vi "3phase PLL.vi"(0 "A":fxp<+/-,32,4>, 1 "wo":dbl, 2 "B":fxp<+/-,32,4>, 3 "C":fxp<+/-,32,4>, 4 "dt (s)":dbl=-1.0 format="%.3f", 5 "PID gains":T1={"proportional gain (Kc)"=1.0, "integral time (Ti, min)"=0.01, "derivative time (Td, min)"=0.0} {"derivative time (Td, min)" format="%.3f"; "integral time (Ti, min)" format="%.3f"; "proportional gain (Kc)" format="%.3f"}) -> (6 "Frequency":dbl, 7 "Phase":dbl)   [LabVIEW 2016]
uses:
  <vilib>/addons/control/pid/pid.llb/PID (DBL).vi
  <vilib>/addons/control/pid/NI_PID_pid.lvlib
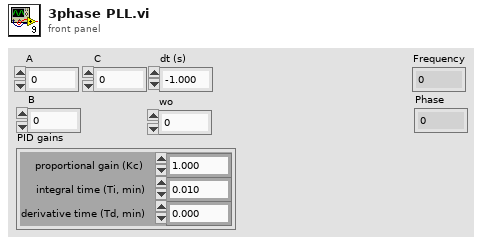
[diagram p1: front panel]
types:
  T1 = cluster{"proportional gain (Kc)":dbl, "integral time (Ti, min)":dbl, "derivative time (Td, min)":dbl}
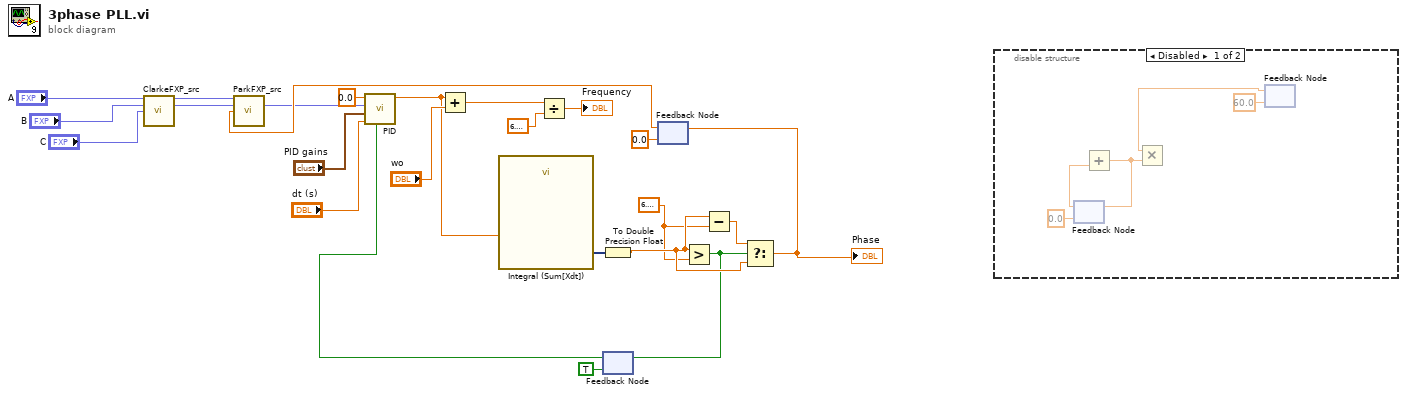
[diagram p0: block diagram]
diagram:
  w9 = 6.283185307179586
  n1 = call "ClarkeFXP_src.vi"("A"="A", "B"="B", "C"="C") -> ("alpha"=w24:fxp<+/-,32,4>, "beta"=w23:fxp<+/-,32,4>)  [unwired: 11 in]
  n2 = feedback #1(TRUE) -> (w2:bool)
  n3 = feedback #2(0.0) -> (w16:dbl)
  n4 = call "ParkFXP_src.vi"("alpha"=w24, "beta"=w23, "theta"=w16) -> ("quadrature"=w5:fxp<+/-,32,4>)  [unwired: 11 in, 1 out]
  n5 = call-poly <vilib>:"PID.vi"("reinitialize? (F)"=w2, "dt (s)"="dt (s)", "PID gains"="PID gains", "process variable"=w5, "setpoint"=0.0) -> ("output"=w6:dbl)  [unwired: 5 in, 1 out]
  n6 = Add(x=w6, y="wo") -> (x+y=w13:dbl)
  n7 = call "Integral (Sum[Xdt])"("Signals"=w6) -> ("Result"=w14:dynamicdata)  [unwired: 5 in, 1 out]
  n8 = Divide(x=w13, y=6.283185307179586) -> (x/y=→"Frequency":dbl)
  n9 = To Double Precision Float(number=w14) -> (double precision float=w10:dbl)
  n10 = Greater?(x=w10, y=w9) -> (0:w3:bool)
  n11 = feedback-in #1(w3) -> ()
  n12 = Subtract(x=w10, y=w9) -> (x-y=w11:dbl)
  n13 = Select(t=w11, s=w3, f=w10) -> (s? t:f=w8:dbl)
  "Phase" <- w8
  n14 = feedback-in #2(w8) -> ()
  n15 = disable-structure shown="Disabled" {
    frame Disabled {
      n16 = feedback #3(0.0) -> (w29:dbl)
      n17 = Add(y=w29) -> (x+y=w25:dbl)  [unwired: 1 in]
      n18 = feedback-in #3(w25) -> ()
      n19 = feedback #4(60.0) -> (w26:dbl)
      n20 = Multiply(x=w26, y=w25) -> ()  [unwired: 1 out]
      n21 = feedback-in #4() -> ()  [unwired: 1 out]
    }
    frame Enabled {
    }
  }
